vi "Edit Config.vi"(8 "error in (no error)":errorcluster, 11 "General Parser in":refnum<class "General Parser.lvclass">) -> (0 "error out":errorcluster, 3 "General Parser out":refnum<class "General Parser.lvclass">)   [LabVIEW 2018, in "General Parser.lvclass"]
doc: "General Parser.lvclass:Edit Config.vi\n\nThis VI is used to edit the General Parser configuration parameters.\n\nInstrument Communication Module Version 1.0\nSeptember, 2017 Original Code Consulting David Thomson\n www.originalcode.com"
uses:
  General Parser.lvclass
  General Parser Config.ctl
  Controls/ICM Class Editor State.ctl
  Controls/ICM Editor Command.ctl
  General Parser.lvclass/General Parser.ctl
panel:
  in  "Test":bool
  in  "Flash Save":bool
  in  "Save":bool
  in  "Revert":bool
  in  "General Parse Config":T1
  # "The General Parser can be used to parse many data\nstrings using a standard LabVIEW format string. ICM\nalso includes additional formatting functions that are\ndescribed in the documentation."
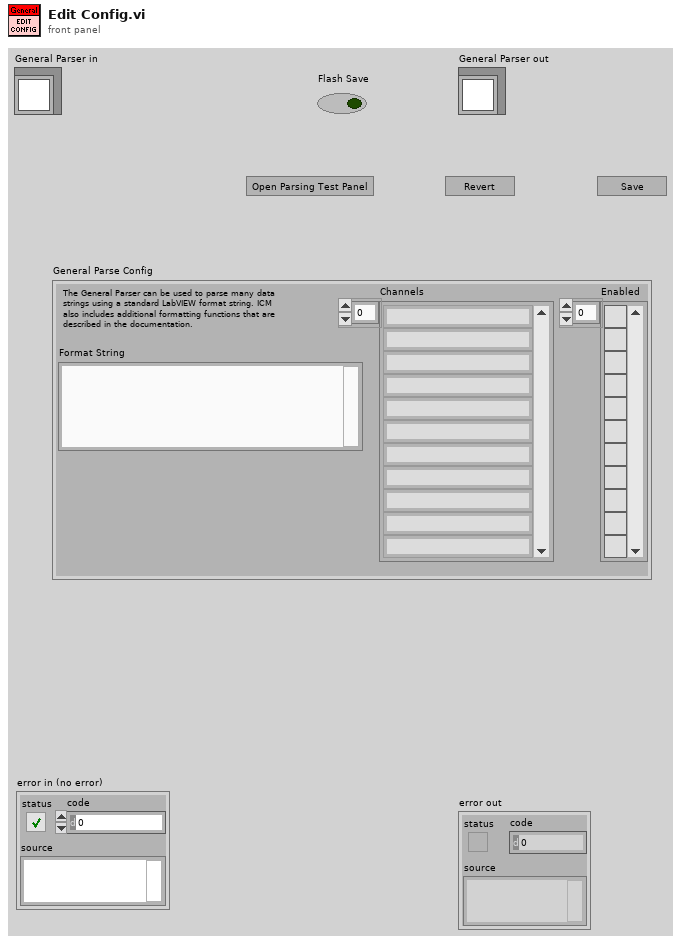
[diagram p1: front panel]
types:
  T1 = typedef "General Parser.lvclass/General Parser Config.ctl" = cluster{"Format String":string, "Channels":string[], "Enabled":bool[]}
  T2 = typedef "ICM Editor Command.ctl" = enum16{"No-op", "Exit"}
  T3 = typedef "ICM Class Editor State.ctl" = enum16{"Init", "Wait", "Write", "Read", "Display", "Set Flashing", "Error", "Stop"}
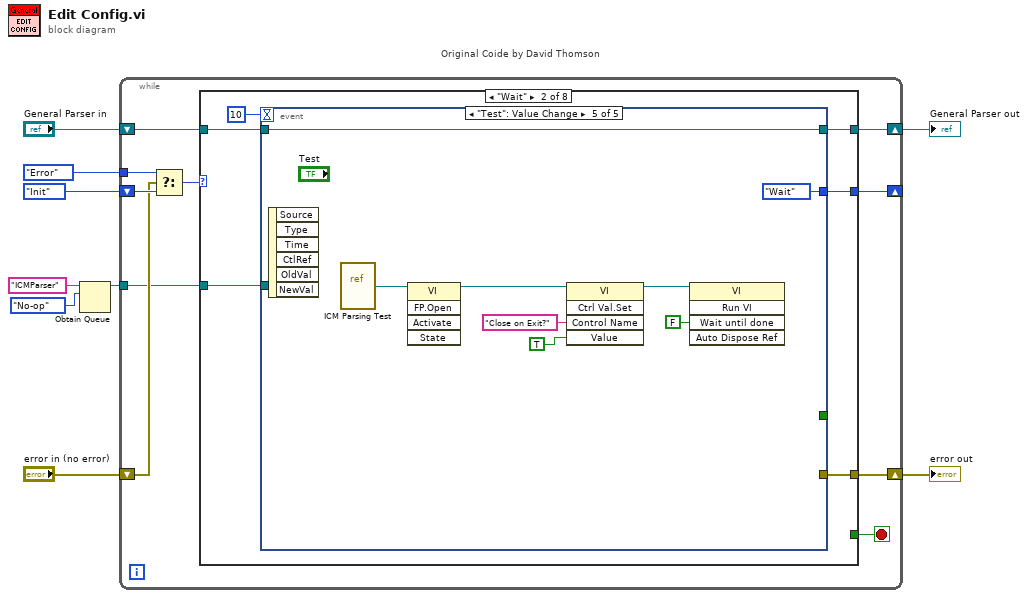
[diagram p0: block diagram]
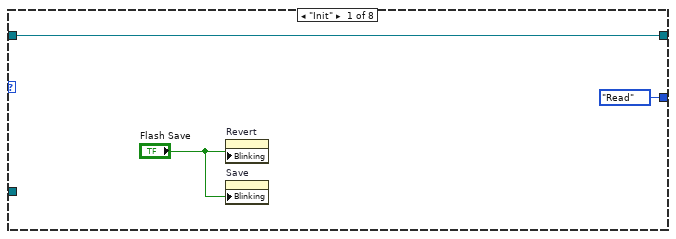
[diagram p2: hidden frame]
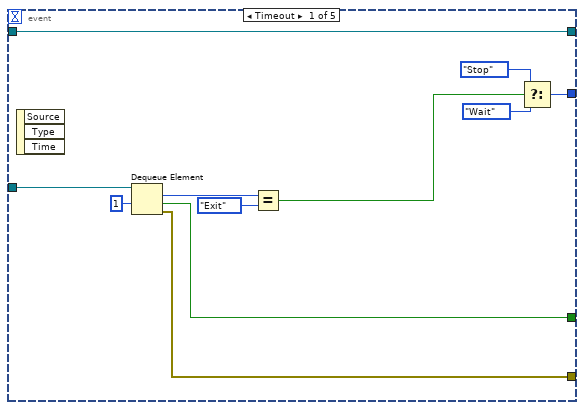
[diagram p3: hidden frame]
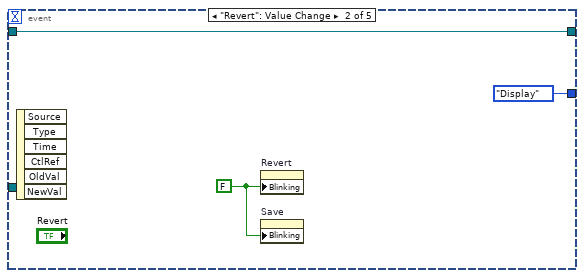
[diagram p4: hidden frame]
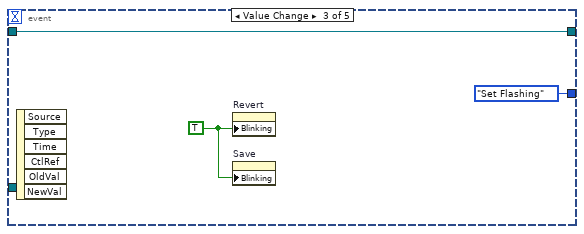
[diagram p5: hidden frame]
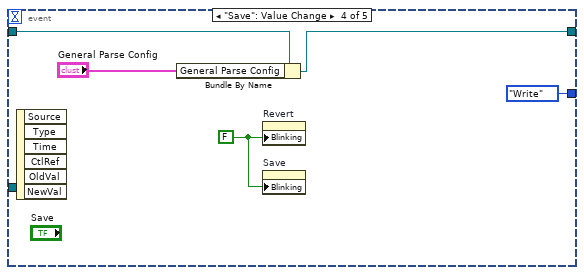
[diagram p6: hidden frame]
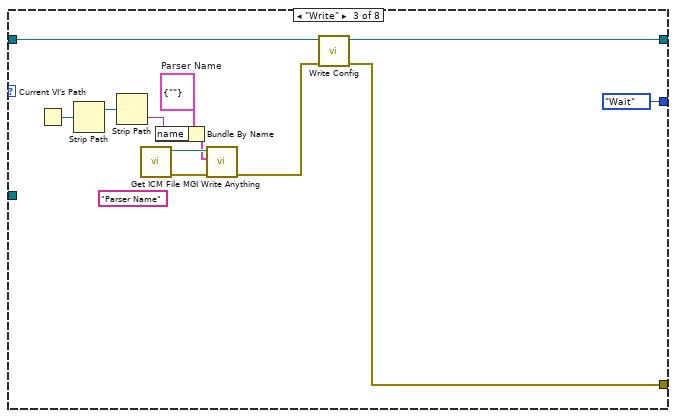
[diagram p7: hidden frame]
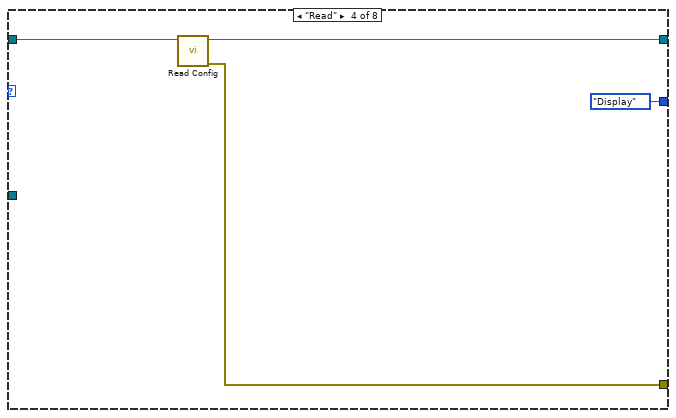
[diagram p8: hidden frame]
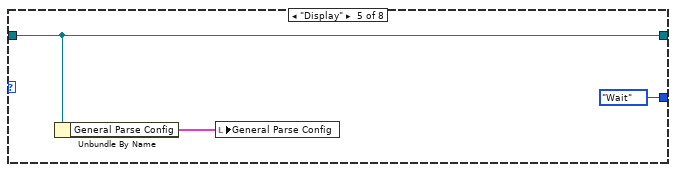
[diagram p9: hidden frame]
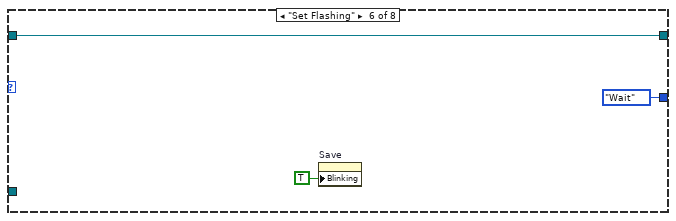
[diagram p10: hidden frame]
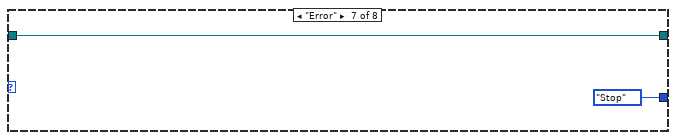
[diagram p11: hidden frame]
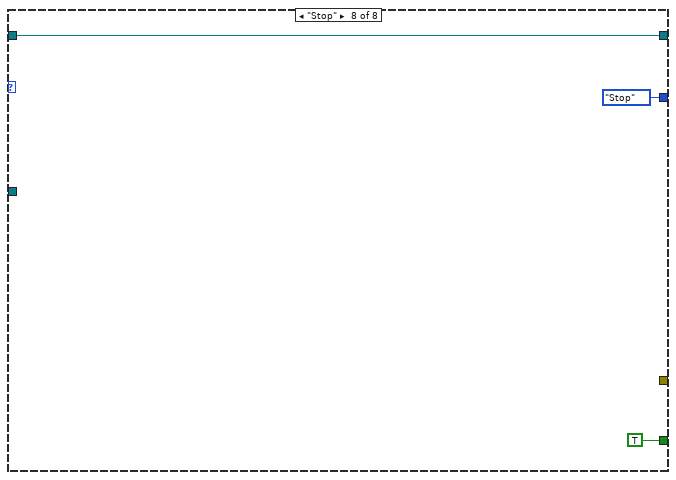
[diagram p12: hidden frame]
diagram:
  n1 = Obtain Queue(name (unnamed)="ICMParser", element data type=ICM_Editor_Command."No-op" ("Editor Command")) -> (queue out=w1:refnum<queue>)  [unwired: 3 in, 2 out]
  n2 = while "Original Coide by David Thomson" {
    shift-right: [w19] -> w8
    shift-left: "General Parser in" -> [w18]
    shift-right: [w12] -> _
    shift-left: ICM_Class_Editor_State."Init" ("Config State") -> [w16]
    shift-right: [w11] -> w6
    shift-left: "error in (no error)" -> [w14]
    tunnel: ICM_Class_Editor_State."Error" ("Config State") -> [w13]
    tunnel: w1 -> [w10]
    stop <- w17 stop-if-true
    n3 = Select(t=w13, s=w14, f=w16) -> (s? t:f=w15:T3)
    n4 = case shown="\"Wait\"" w15 {
      tunnel: [w21 w26 w68 w72 w77 w80 w82 w85] -> w19
      tunnel: w18 -> [w21 w25 w69 w74 w77 w80 w82 w85]
      tunnel: [_ _ _ _ _ _ _ TRUE] -> w17
      tunnel: [ICM_Class_Editor_State."Read" ("Config State") w27 ICM_Class_Editor_State."Wait" ("Config State") ICM_Class_Editor_State."Display" ("Config State") ICM_Class_Editor_State."Wait" ("Config State") ICM_Class_Editor_State."Wait" ("Config State") ICM_Class_Editor_State."Stop" ("Config State") ICM_Class_Editor_State."Stop" ("Config State")] -> w12
      tunnel: [_ w23 w67 w73 _ _ _ _] -> w11
      tunnel: w10 -> [_ w24 _ _ _ _ _ _]
      frame "Init" {
        n5 = property on="Revert" class="Bool"("Blinking"="Flash Save") -> ()  [unwired: 2 in, 2 out]
        n6 = property on="Save" class="Bool"("Blinking"="Flash Save") -> ()  [unwired: 2 in, 2 out]
      }
      frame "Wait" {
        n7 = event shown="[4] \"Test\": Value Change" {
          selector: _ -> [_ _ _ _ _]
          dyn-events: _ -> [_ _ _ _ _]
          timeout: 10 -> [_ _ _ _ _]
          tunnel: [w36 ICM_Class_Editor_State."Display" ("Config State") ICM_Class_Editor_State."Set Flashing" ("Config State") ICM_Class_Editor_State."Write" ("Config State") ICM_Class_Editor_State."Wait" ("Config State")] -> w27
          tunnel: [w39 w41 w45 w47 w58] -> w26
          tunnel: w25 -> [w39 w41 w45 w48 w58]
          tunnel: w24 -> [w38 _ _ _ _]
          tunnel: [w30 _ _ _ _] -> w23
          tunnel: [w29 _ _ _ _] -> _
          event Timeout {
            n8 = event-data() -> ()  [unwired: 1 in, 3 out]
            n9 = Dequeue Element(queue=w38, timeout in ms (-1)=1) -> (element=w35:T2, timed out?=w29:bool, error out=w30:errorcluster)  [unwired: 1 in, 1 out]
            n10 = Equal?(x=w35, y=ICM_Editor_Command."Exit") -> (x = y?=w33:bool)
            n11 = Select(t=ICM_Class_Editor_State."Stop" ("Config State"), s=w33, f=ICM_Class_Editor_State."Wait" ("Config State")) -> (s? t:f=w36:T3)
          }
          event "Revert": Value Change {
            w40 = FALSE ("Blinking")
            n12 = event-data() -> ()  [unwired: 1 in, 6 out]
            n13 = property on="Revert" class="Bool"("Blinking"=w40) -> ()  [unwired: 2 in, 2 out]
            n14 = property on="Save" class="Bool"("Blinking"=w40) -> ()  [unwired: 2 in, 2 out]
          }
          event Value Change {
            w43 = TRUE ("Blinking")
            n15 = event-data() -> ()  [unwired: 1 in, 6 out]
            n16 = property on="Revert" class="Bool"("Blinking"=w43) -> ()  [unwired: 2 in, 2 out]
            n17 = property on="Save" class="Bool"("Blinking"=w43) -> ()  [unwired: 2 in, 2 out]
          }
          event "Save": Value Change {
            w46 = FALSE ("Blinking")
            n18 = event-data() -> ()  [unwired: 1 in, 6 out]
            n19 = Bundle By Name(cluster=w48, "General Parse Config"="General Parse Config") -> (w47:refnum<class "General Parser.lvclass">)
            n20 = property on="Revert" class="Bool"("Blinking"=w46) -> ()  [unwired: 2 in, 2 out]
            n21 = property on="Save" class="Bool"("Blinking"=w46) -> ()  [unwired: 2 in, 2 out]
          }
          event "Test": Value Change {
            n22 = event-data() -> ()  [unwired: 1 in, 6 out]
            n23 = vi-ref "ICM Parsing Test.vi"() -> (w56:refnum<vi>)
            n24 = invoke class="VI" method="FP.Open"(reference=w56) -> (reference out=w54:refnum<vi>)  [unwired: 4 in, 4 out]
            n25 = invoke class="VI" method="Ctrl Val.Set"(reference=w54, "Control Name"="Close on Exit?", "Value"=TRUE) -> (reference out=w53:refnum<vi>)  [unwired: 2 in, 4 out]
            n26 = invoke class="VI" method="Run VI"(reference=w53, "Wait until done"=FALSE ("Wait Until Done")) -> ()  [unwired: 3 in, 5 out]
          }
        }
      }
      frame "Write" {
        w59 = cluster{"name":string} {"name"=""}  # Parser Name
        (unwired) "Parser Name" ("Section Name (Name of \"Anything\")")
        n27 = Current VI's Path() -> (path=w66:path)
        n28 = Strip Path(path=w66) -> (stripped path=w65:path)  [unwired: 1 out]
        n29 = Strip Path(path=w65) -> (name=w60:string)  [unwired: 1 out]
        n30 = call "Get ICM File.vi"() -> ("error out"=w63:errorcluster, "ICM File"=w64:path)  [unwired: 10 in]
        n31 = Bundle By Name(cluster=w59, "name"=w60) -> (w61:cluster{"name":string})
        n32 = call <userlib>:"MGI Write Anything.vi"("Error In"=w63, "Anything"=w61, "Path (dialog)"=w64) -> ("Error Out"=w62:errorcluster)  [unwired: 6 in, 2 out]
        n33 = call-dynamic "Write Config.vi"("error in (no error)"=w62, "General Parser in"=w69) -> ("error out"=w67:errorcluster, "General Parser out"=w68:refnum<class "General Parser.lvclass">)  [unwired: 8 in]
      }
      frame "Read" {
        n34 = call-dynamic "Read Config.vi"("General Parser in"=w74) -> ("error out"=w73:errorcluster, "General Parser out"=w72:refnum<class "General Parser.lvclass">)  [unwired: 9 in]
      }
      frame "Display" {
        n35 = Unbundle By Name(w77) -> ("General Parse Config"=w76:T1)
        n36 = local write "General Parse Config"(w76) -> ()
      }
      frame "Set Flashing" {
        n37 = property on="Save" class="Bool"("Blinking"=TRUE) -> ()  [unwired: 2 in, 2 out]
      }
      frame "Error" {
      }
      frame "Stop" {
      }
    }
  }
  "error out" <- w6
  "General Parser out" <- w8
